vi "Get Async FIFO Refs.vi"(8 "error in (no error)":errorcluster, 10 "Data Access API In":refnum<class "Data Access Engine.lvclass">, 11 "Async State Vars In":T1) -> (0 "error out":errorcluster, 2 "Data Access API Out":refnum<class "Data Access Engine.lvclass">, 3 "Async State Vars Out":T1)   [LabVIEW 2015, in "Waveform-Processing-Custom-Device Engine.lvlib"]
uses:
  Waveform-Processing-Custom-Device Engine.lvlib
  Types/AsyncStateVariables.ctl
  <vilib>/NI Veristand/Custom Device Waveform API/Single Waveform Read (DBL)/Single Waveform Read (DBL).lvclass
  <vilib>/NI Veristand/Custom Device Waveform API/Single Waveform Write (DBL)/Single Waveform Write (DBL).lvclass
  <vilib>/NI Veristand/Custom Device API/Waveform Data Reference.ctl
  <vilib>/NI/NIVS Inline Async API/_Data Access Engine/Data Access Engine/Types/Write.DVR.ctl
  <vilib>/NI/NIVS Inline Async API/_Data Access Engine/Access Type Classes/Write/Write.lvclass
  <vilib>/NI/NIVS Inline Async API/_Data Access Engine/Data Access Engine/Types/Read.DVR.ctl
  <vilib>/NI/NIVS Inline Async API/_Data Access Engine/Access Type Classes/Read/Read.lvclass
  <vilib>/NI/NIVS Inline Async API/_Data Access Engine/Data Access Engine/Data Access Engine.lvclass
  Shared/Constants.vi
  <vilib>/NI/NIVS Inline Async API/_Data Access Engine/Data Access Engine/Methods/Write.Lookup.vi
  <vilib>/NI/NIVS Inline Async API/_Data Access Engine/Data Access Engine/Methods/Read.Lookup.vi
  Shared/Waveform-Processing-Custom-Device Shared.lvlib
  <vilib>/NI VeriStand/Custom Device API/Custom Device API.lvlib
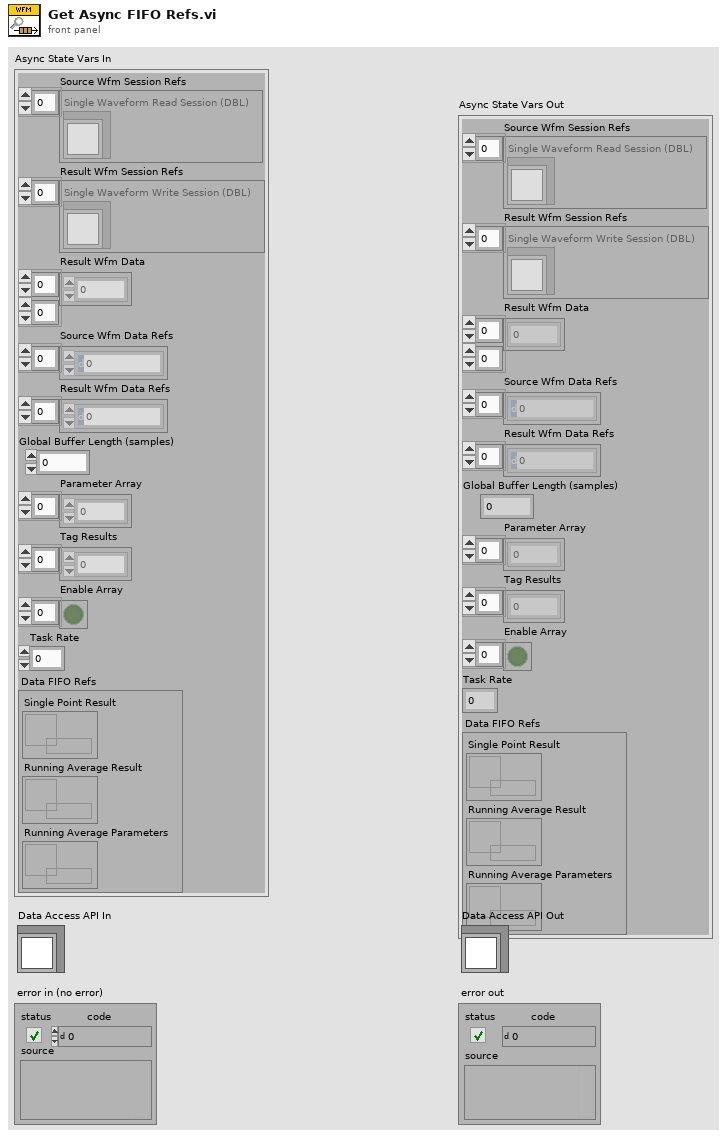
[diagram p1: front panel]
types:
  T1 = typedef "Waveform-Processing-Custom-Device Engine.lvlib/AsyncStateVariables.ctl" = cluster{"Source Wfm Session Refs":refnum<class "Single Waveform Read (DBL).lvclass">[], "Result Wfm Session Refs":refnum<class "Single Waveform Write (DBL).lvclass">[], "Result Wfm Data":dbl[][], "Source Wfm Data Refs":T2[], "Result Wfm Data Refs":T2[], "Global Buffer Length (samples)":dbl, "Parameter Array":dbl[], "Tag Results":dbl[], "Enable Array":bool[], "Task Rate":dbl, "Data FIFO Refs":cluster{"Single Point Result":T3, "Running Average Result":T3, "Running Average Parameters":T4}}
  T2 = typedef "Custom Device API.lvlib/Waveform Data Reference.ctl" = i32
  T3 = typedef "Data Access Engine.lvlib/Data Access Engine.lvclass/Write.DVR.ctl" = refnum<data-value>
  T4 = typedef "Data Access Engine.lvlib/Data Access Engine.lvclass/Read.DVR.ctl" = refnum<data-value>
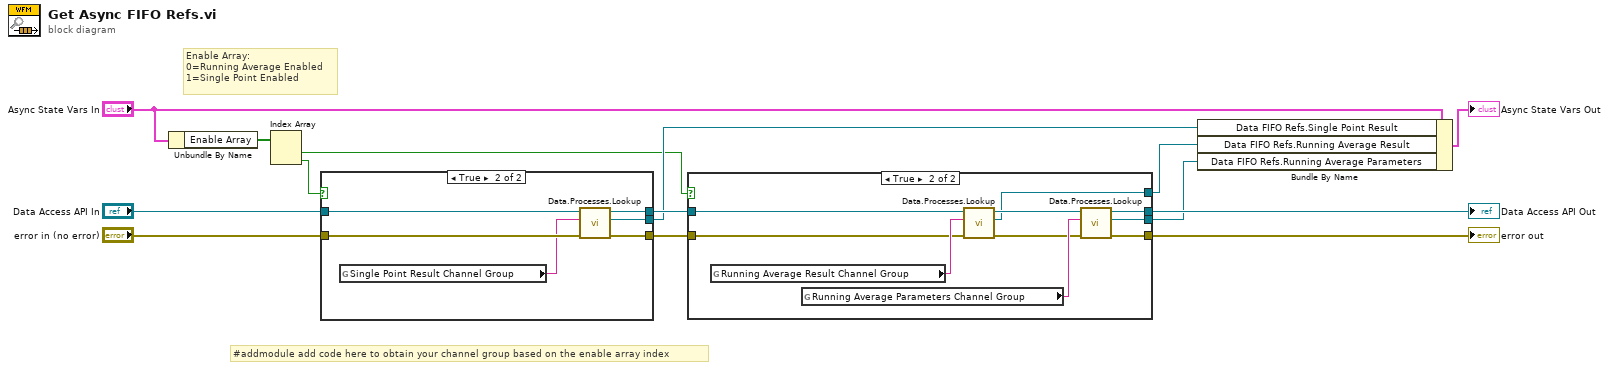
[diagram p0: block diagram]
diagram:
  # "#addmodule add code here to obtain your channel group based on the enable array index"
  # "Enable Array:\n0=Running Average Enabled\n1=Single Point Enabled"
  n1 = Unbundle By Name("Async State Vars In") -> ("Enable Array"=w5:bool[])
  n2 = Index Array(array=w5) -> (element #1=w1:bool, element #2=w4:bool)  [unwired: 2 in]
  n3 = case shown="True" w4 {
    tunnel: "Data Access API In" -> [w16 w22]
    tunnel: [w16 w21] -> w11
    tunnel: "error in (no error)" -> [w15 w20]
    tunnel: [_ w19] -> w8
    tunnel: [w15 w17] -> w3
    frame False {
      # "If single point is not enabled, pass data through\nand create default refnum for FIFO"
    }
    frame True {
      n4 = global read "Constants.vi" "Single Point Result Channel Group"() -> (w18:string)
      n5 = call-poly <vilib>:"Data.Processes.Lookup.vi"("error in (no error)"=w20, "Name"=w18, "Data Access API in"=w22) -> ("error out"=w17:errorcluster, "Ref"=w19:T3, "Data Access API out"=w21:refnum<class "Data Access Engine.lvclass">)  [unwired: 5 in, 1 out]
    }
  }
  n6 = case shown="True" w1 {
    tunnel: [w23 w33] -> w14
    tunnel: w11 -> [w23 w32]
    tunnel: [_ w31] -> w9
    tunnel: [w24 w27] -> w7
    tunnel: w3 -> [w24 w26]
    tunnel: [_ w25] -> w2
    frame False {
      # "If running average is not enabled, pass data through\nand create default refnum for both FIFOs"
    }
    frame True {
      n7 = global read "Constants.vi" "Running Average Result Channel Group"() -> (w30:string)
      n8 = global read "Constants.vi" "Running Average Parameters Channel Group"() -> (w29:string)
      n9 = call-poly <vilib>:"Data.Processes.Lookup.vi"("error in (no error)"=w26, "Name"=w30, "Data Access API in"=w32) -> ("error out"=w28:errorcluster, "Ref"=w25:T3, "Data Access API out"=w34:refnum<class "Data Access Engine.lvclass">)  [unwired: 5 in, 1 out]
      n10 = call-poly <vilib>:"Data.Processes.Lookup.vi"("error in (no error)"=w28, "Name"=w29, "Data Access API in"=w34) -> ("error out"=w27:errorcluster, "Ref"=w31:T4, "Data Access API out"=w33:refnum<class "Data Access Engine.lvclass">)  [unwired: 5 in, 1 out]
    }
  }
  "error out" <- w7
  "Data Access API Out" <- w14
  n11 = Bundle By Name(cluster="Async State Vars In", "Data FIFO Refs.Single Point Result"=w8, "Data FIFO Refs.Running Average Result"=w2, "Data FIFO Refs.Running Average Parameters"=w9) -> (→"Async State Vars Out":T1)
